vi "Primary Xbox Drive.vi"(10 "Primary":T3={"Buttons"={"A"=FALSE, "B"=FALSE, "X"=FALSE, "Y"=FALSE, "Left Bumper"=FALSE, "Right Bumper"=FALSE, "Back"=FALSE, "Start"=FALSE, "Left Thumbstick"=FALSE, "Right Thumbstick"=FALSE}, "Axes"={"Left Stick X "=0.0, "Left Stick Y"=0.0, "Triggers"=-0.0, "Right Stick X"=0.0, "Right Stick Y"=0.0, "D-Pad X"=0.0}}, 11 "Dash Data":T2={"Joy Stick"={"Primary"={"Buttons"={"A"=FALSE, "B"=FALSE, "X"=FALSE, "Y"=FALSE, "Left Bumper"=FALSE, "Right Bumper"=FALSE, "Back"=FALSE, "Start"=FALSE, "Left Thumbstick"=FALSE, "Right Thumbstick"=FALSE}, "Axes"={"Left Stick X "=0.0, "Left Stick Y"=0.0, "Triggers"=-0.0, "Right Stick X"=0.0, "Right Stick Y"=0.0, "D-Pad X"=0.0}}, "Secondary"={"Buttons"={"A"=FALSE, "B"=FALSE, "X"=FALSE, "Y"=FALSE, "Left Bumper"=FALSE, "Right Bumper"=FALSE, "Back"=FALSE, "Start"=FALSE, "Left Thumbstick"=FALSE, "Right Thumbstick"=FALSE}, "Axes"={"Left Stick X "=0.0, "Left Stick Y"=0.0, "Triggers"=0.0, "Right Stick X"=0.0, "Right Stick Y"=0.0, "D-Pad X"=0.0}}}, "Shooter"={"RPM Current"=0.0, "RPM Set"=0.0, "In Range?"=FALSE}, "Arm"={"Arm Current"=0.0, "Arm Set"=0.0, "At Position?"=FALSE, "Reset Encoder"=FALSE}, "Drive"={"Right"=0.0, "Left"=0.0}, "Climb State"=enum."Arm Attach", "Change Retical"=FALSE, "Solenoids"={"Robot Angle"=enum."Off", "Shooter Angle"=enum."Off", "Arm Lock"=enum."Off"}, "Shooter Speeds"=[]}) -> (3 "Dash Data Out":T2={"Joy Stick"={"Primary"={"Buttons"={"A"=FALSE, "B"=FALSE, "X"=FALSE, "Y"=FALSE, "Left Bumper"=FALSE, "Right Bumper"=FALSE, "Back"=FALSE, "Start"=FALSE, "Left Thumbstick"=FALSE, "Right Thumbstick"=FALSE}, "Axes"={"Left Stick X "=0.0, "Left Stick Y"=0.0, "Triggers"=-0.0, "Right Stick X"=0.0, "Right Stick Y"=0.0, "D-Pad X"=0.0}}, "Secondary"={"Buttons"={"A"=FALSE, "B"=FALSE, "X"=FALSE, "Y"=FALSE, "Left Bumper"=FALSE, "Right Bumper"=FALSE, "Back"=FALSE, "Start"=FALSE, "Left Thumbstick"=FALSE, "Right Thumbstick"=FALSE}, "Axes"={"Left Stick X "=0.0, "Left Stick Y"=0.0, "Triggers"=0.0, "Right Stick X"=0.0, "Right Stick Y"=0.0, "D-Pad X"=0.0}}}, "Shooter"={"RPM Current"=0.0, "RPM Set"=0.0, "In Range?"=FALSE}, "Arm"={"Arm Current"=0.0, "Arm Set"=0.0, "At Position?"=FALSE, "Reset Encoder"=FALSE}, "Drive"={"Right"=0.0, "Left"=0.0}, "Climb State"=enum."Arm Attach", "Change Retical"=FALSE, "Solenoids"={"Robot Angle"=enum."Off", "Shooter Angle"=enum."Off", "Arm Lock"=enum."Off"}, "Shooter Speeds"=[]})   [LabVIEW 2012]
uses:
  <vilib>/Rock Robotics/WPI/Solenoid/WPI_SolenoidValue.ctl
types:
  T1 = typedef "WPI_SolenoidValue.ctl" = enum16{"Off", "On", "Forward", "Reverse"}
  T2 = cluster{"Joy Stick":cluster{"Primary":cluster{"Buttons":cluster{"A":bool, "B":bool, "X":bool, "Y":bool, "Left Bumper":bool, "Right Bumper":bool, "Back":bool, "Start":bool, "Left Thumbstick":bool, "Right Thumbstick":bool}, "Axes":cluster{"Left Stick X ":dbl, "Left Stick Y":dbl, "Triggers":dbl, "Right Stick X":dbl, "Right Stick Y":dbl, "D-Pad X":dbl}}, "Secondary":cluster{"Buttons":cluster{"A":bool, "B":bool, "X":bool, "Y":bool, "Left Bumper":bool, "Right Bumper":bool, "Back":bool, "Start":bool, "Left Thumbstick":bool, "Right Thumbstick":bool}, "Axes":cluster{"Left Stick X ":dbl, "Left Stick Y":dbl, "Triggers":dbl, "Right Stick X":dbl, "Right Stick Y":dbl, "D-Pad X":dbl}}}, "Shooter":cluster{"RPM Current":dbl, "RPM Set":dbl, "In Range?":bool}, "Arm":cluster{"Arm Current":dbl, "Arm Set":dbl, "At Position?":bool, "Reset Encoder":bool}, "Drive":cluster{"Right":dbl, "Left":dbl}, "Climb State":enum16{"Arm Wait", "Arm Up", "Arm Down", "Arm Attach"}, "Change Retical":bool, "Solenoids":cluster{"Robot Angle":T1, "Shooter Angle":T1, "Arm Lock":T1}, "Shooter Speeds":dbl[]}
  T3 = cluster{"Buttons":cluster{"A":bool, "B":bool, "X":bool, "Y":bool, "Left Bumper":bool, "Right Bumper":bool, "Back":bool, "Start":bool, "Left Thumbstick":bool, "Right Thumbstick":bool}, "Axes":cluster{"Left Stick X ":dbl, "Left Stick Y":dbl, "Triggers":dbl, "Right Stick X":dbl, "Right Stick Y":dbl, "D-Pad X":dbl}}
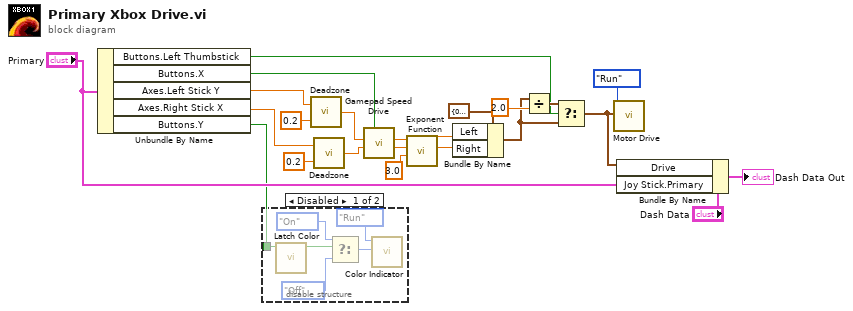
[diagram p0: block diagram]
diagram:
  n1 = Unbundle By Name("Primary") -> ("Buttons.Left Thumbstick"=w2:bool, "Buttons.X"=w5:bool, "Axes.Left Stick Y"=w4:dbl, "Axes.Right Stick X"=w3:dbl, "Buttons.Y"=w1:bool)
  n2 = disable-structure shown="Disabled" {
    disable-tunnel: w1 -> [w29 _]
    frame Disabled {
      n3 = call "Latch Color.vi"("Input"=w29) -> ("Latched"=w28:bool)  [unwired: 10 in]
      n4 = Select(t=WPI_SolenoidValue."On" ("Value"), s=w28, f=WPI_SolenoidValue."Off" ("Value")) -> (s? t:f=w25:T1)
      n5 = call "Color Indicator.vi"("Value"=w25, "Enum"=enum16{"Start", "Run", "End"}."Run") -> ()  [unwired: 10 in]
    }
    frame Enabled {
    }
  }
  n6 = call "Deadzone.vi"("Deadzone"=0.2, "Input"=w4) -> ("Output"=w15:dbl)
  n7 = call "Deadzone.vi"("Deadzone"=0.2, "Input"=w3) -> ("Output"=w13:dbl)
  n8 = call "Gamepad Speed Drive.vi"("Quick Turn"=w5, "Turn"=w13, "Speed"=w15) -> ("Right Output"=w18:dbl, "Left Output"=w19:dbl)  [unwired: 7 in]
  n9 = call "Exponent Function.vi"("Exponent"=3.0, "Left In"=w18, "Right In"=w19) -> ("Right Out"=w10:dbl, "Left Out"=w11:dbl)  [unwired: 7 in]
  n10 = Bundle By Name(cluster=cluster{"Right":dbl, "Left":dbl} {"Right"=0.0, "Left"=0.0} ("Motor"), "Left"=w11, "Right"=w10) -> (w8:cluster{"Right":dbl, "Left":dbl})
  n11 = Divide(x=w8, y=2.0) -> (x/y=w7:cluster{"Right":dbl, "Left":dbl})
  n12 = Select(t=w7, s=w2, f=w8) -> (s? t:f=w6:cluster{"Right":dbl, "Left":dbl})
  n13 = call "Motor Drive.vi"("Motor"=w6, "Enum"=enum16{"Start", "Run", "End"}."Run") -> ()  [unwired: 10 in]
  n14 = Bundle By Name(cluster="Dash Data", "Drive"=w6, "Joy Stick.Primary"="Primary") -> (→"Dash Data Out":T2)
